vi "timeout error fg.vi"(2 "Location":T1="Auto_3", 3 "Timeout Error?":bool) -> (0 "# of Timeouts":u32, 1 "Time Out Error This Match":bool)   [LabVIEW 2013]
uses:
  typedefs/location of error.ctl
panel:
  # "A Funtctional Global to Store if there has been a Timeout Error"
  # "Very unlike a usual FG"
  # "It writes true if the timeout error control is true,\nbut if it is false it does nothing. This causes a permanent\ntime out error output, which is good, it also displays how\nmany there have been."
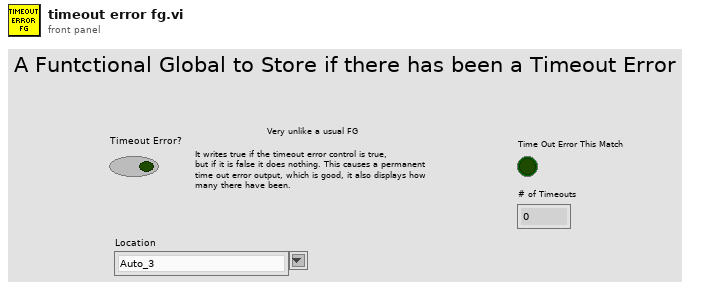
[diagram p1: front panel]
types:
  T1 = typedef "location of error.ctl" = string
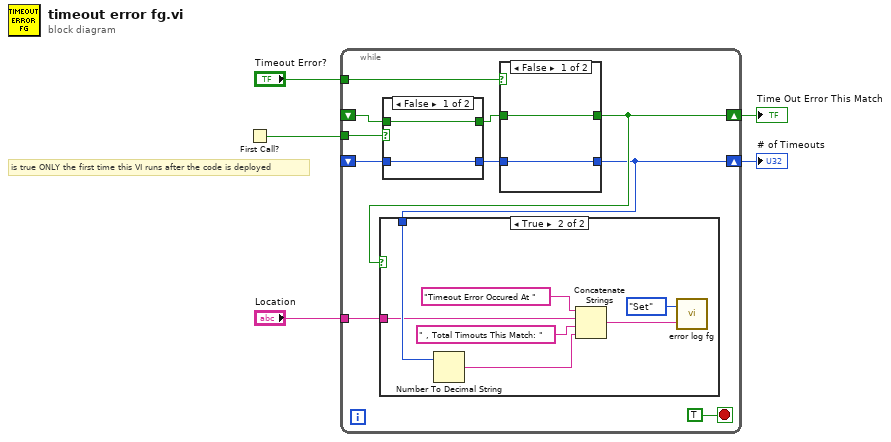
[diagram p0: block diagram]
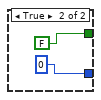
[diagram p3: hidden frame]
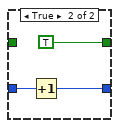
[diagram p4: hidden frame]
diagram:
  # "is true ONLY the first time this VI runs after the code is deployed"
  n1 = First Call?() -> (First Call?: T/F=w2:bool)
  n2 = while {
    shift-right: [w8] -> w4
    shift-left: _ -> [w13]
    tunnel: "Timeout Error?" -> [w14]
    shift-right: [w7] -> w3
    shift-left: _ -> [w11]
    tunnel: w2 -> [w9]
    tunnel: "Location" -> [w6]
    stop <- TRUE stop-if-true
    n3 = case shown="False" w9 {
      tunnel: w13 -> [w24 _]
      tunnel: [w24 FALSE] -> w12
      tunnel: w11 -> [w23 _]
      tunnel: [w23 u32 0] -> w10
      frame False {
      }
      frame True {
      }
    }
    n4 = case shown="False" w14 {
      tunnel: [w28 TRUE] -> w8
      tunnel: w12 -> [w28 _]
      tunnel: [w27 w29] -> w7
      tunnel: w10 -> [w27 w30]
      frame False {
      }
      frame True {
        n5 = Increment(x=w30) -> (x+1=w29:u32)
      }
    }
    n6 = case shown="True" w8 {
      tunnel: w7 -> [_ w21]
      tunnel: w6 -> [_ w19]
      frame False {
      }
      frame True {
        n7 = Number To Decimal String(number=w21) -> (decimal integer string=w17:string)  [unwired: 1 in]
        n8 = Concatenate Strings("Timeout Error Occured At ", w19, " , Total Timouts This Match: ", w17) -> (w16:string)
        n9 = call "error log fg.vi"("Error"=w16, "Log Mode"=enum16{"Get", "Set", "Clear"}."Set") -> ()  [unwired: 2 out]
      }
    }
  }
  "Time Out Error This Match" <- w4
  "# of Timeouts" <- w3
